vi "CONV 1D Integer Array to String.vi"(0 "1-D Integer":i32[](array[numeric]), 1 "Delimiter (,)":string=",") -> (6 "String":string)   [LabVIEW 2017]
doc: "This routine converts a 1-D Numeric Array into a string list. The delimiter may be one or more characters."
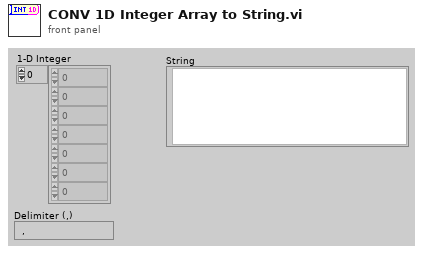
[diagram p1: front panel]
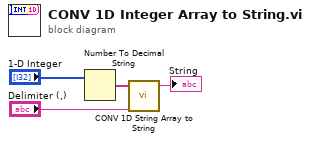
[diagram p0: block diagram]
diagram:
  n1 = Number To Decimal String(number="1-D Integer") -> (decimal integer string=w3:string[])  [unwired: 1 out]
  n2 = call "CONV 1D String Array to String.vi"("1-D String"=w3, "Delimiter (,)"="Delimiter (,)") -> ("String"=→"String":string)  [unwired: 7 out]
